vi "Initialize Front Panel.vi"(8 "error in (no error)":errorcluster, 11 "ViewManagerDefaultLayout in":refnum<class "ViewManagerDefaultLayout.lvclass">) -> (0 "error out":errorcluster, 3 "ViewManagerDefaultLayout out":refnum<class "ViewManagerDefaultLayout.lvclass">)   [LabVIEW 2017, in "ViewManagerDefaultLayout.lvclass"]
doc: "<License>\nCopyright © 2017 Composed Systems, LLC | All rights reserved\nwww.composed.io\n\nAuthor: Ethan Stern <ethan.stern@composed.io>\n\nThis software is provided \"AS IS\" WITHOUT WARRANTIES, either express or implied, AND IS FOR EDUCATIONAL PURPOSES ONLY.\n</License>MVA Framework 1.7.0.33\nEthan Stern - Composed Systems\nCopyright (c) 2018, Composed Systems"
uses:
  ViewManagerDefaultLayout.lvclass
  C:/Program Files/National Instruments/LabVIEW 2017/vi.lib/Composed/GPM Packages/mva-framework/Source/Framework/IViewManager/IViewManager/IViewManager.lvclass
  mva-viewable/Source/IViewManager/IViewManager/IViewManager.lvclass/IViewManager.ctl
  ViewManagerDefaultLayout.lvclass/ViewManagerDefaultLayout.ctl
  mva-viewable/Source/IViewable/IViewable Messages/Insert Front Panel Msg/Insert Front Panel Msg.lvclass/Insert Front Panel Msg.ctl
  <vilib>/ActorFramework/Message Enqueuer/Message Enqueuer.lvclass/Message Enqueuer.ctl
  <vilib>/ActorFramework/Message Enqueuer/Enqueue.vi
  mva-viewable/Source/IViewable/IViewable Messages/Insert Front Panel Msg/Insert Front Panel Msg.lvclass
  C:/Program Files/National Instruments/LabVIEW 2017/vi.lib/ActorFramework/Message/Message.lvclass
  <vilib>/ActorFramework/Message Priority Queue/Priority Enqueue.vi
  mva-viewable/Source/IViewManager/IViewManager/IViewManager.lvclass
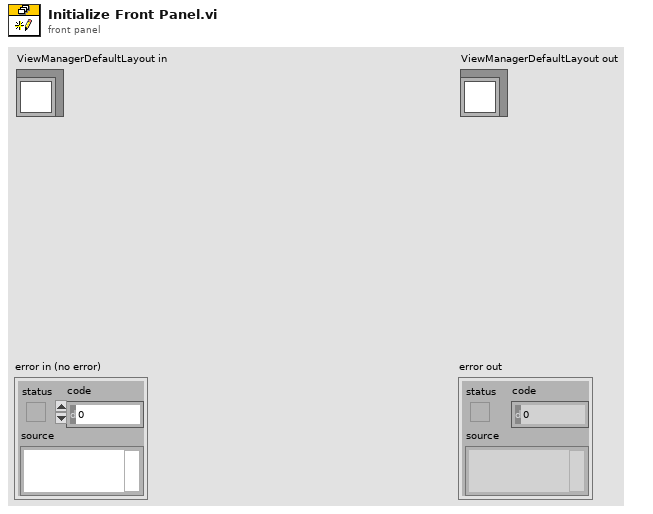
[diagram p1: front panel]
types:
  T1 = typedef "IViewable.lvlib/ProtectedSubpanel.lvclass/Protected Subpanel Reference.ctl" = refnum<data-value>
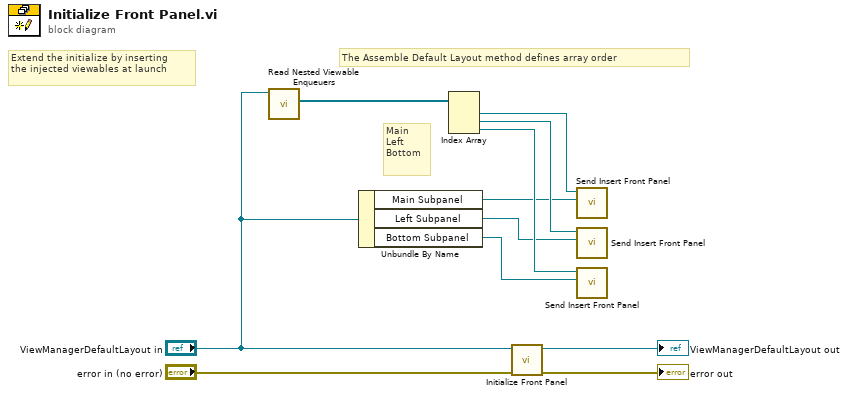
[diagram p0: block diagram]
diagram:
  # "Extend the initialize by inserting\nthe injected viewables at launch"
  # "The Assemble Default Layout method defines array order"
  # "Main\nLeft\nBottom"
  n1 = call "Read Nested Viewable Enqueuers.vi"("IViewManager in"="ViewManagerDefaultLayout in") -> ("Nested Viewable Enqueuers"=w7:refnum<class "Message Enqueuer.lvclass">[])  [unwired: 9 in, 1 out]
  n2 = Unbundle By Name("ViewManagerDefaultLayout in") -> ("Main Subpanel"=w3:T1, "Left Subpanel"=w2:T1, "Bottom Subpanel"=w1:T1)
  n3 = Index Array(array=w7) -> (element #1=w6:refnum<class "Message Enqueuer.lvclass">, element #2=w5:refnum<class "Message Enqueuer.lvclass">, element #3=w4:refnum<class "Message Enqueuer.lvclass">)  [unwired: 3 in]
  n4 = call-parent "Initialize Front Panel.vi"("error in (no error)"="error in (no error)", "IViewable in"="ViewManagerDefaultLayout in") -> ("error out"=→"error out":errorcluster, "IViewable out"=→"ViewManagerDefaultLayout out":refnum<class "ViewManagerDefaultLayout.lvclass">)  [unwired: 8 in]
  n5 = call "Send Insert Front Panel.vi"("Protected Subpanel"=w3, "Message Enqueuer"=w6) -> ()  [unwired: 8 in, 2 out]
  n6 = call "Send Insert Front Panel.vi"("Protected Subpanel"=w2, "Message Enqueuer"=w5) -> ()  [unwired: 8 in, 2 out]
  n7 = call "Send Insert Front Panel.vi"("Protected Subpanel"=w1, "Message Enqueuer"=w4) -> ()  [unwired: 8 in, 2 out]
